vi "Get SecretKey.vi"(8 "error in (no error)":errorcluster, 11 "SMO":refnum<class "SMO.lvclass">) -> (0 "error out":errorcluster, 2 "SecretKey":string, 3 "SMO out":refnum<class "SMO.lvclass">)   [LabVIEW 2021, in "smo.lvlib" / "SMO.lvclass"]
uses:
  SMO.lvclass
  Support/Attribute.Identity/Attribute.Identity.lvclass
  SMO.lvclass/SMO.ctl
  Support/Attribute.Identity/Attribute.Identity.lvclass/Attribute.Identity.ctl
  ReftoDVR--SMO.vi
panel:
  # "For instructions on how to use the JKI State Machine Objects, examples and video tutorials, visit:\nhttp://jki.net/state-machine-objects/\n\nJKI State Machine Objects™\nhttp://jki.net/state-machine-objects/\nCopyright (C) 2005-2015, JKI <info@jki.net>\nALL RIGHTS RESERVED"
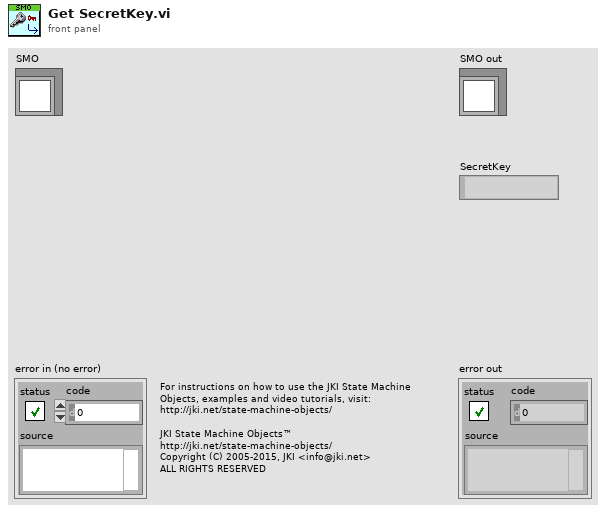
[diagram p1: front panel]
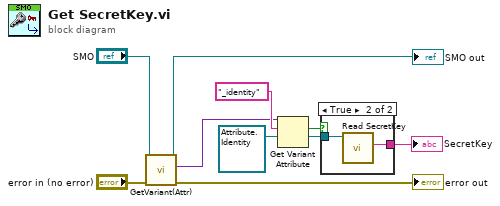
[diagram p0: block diagram]
diagram:
  n1 = call "GetVariant(Attr).vi"("error in (no error)"="error in (no error)", "SMO in"="SMO") -> ("error out"=→"error out":errorcluster, "[Attributes]"=w4:variant, "SMO out"=→"SMO out":refnum<class "SMO.lvclass">)  [unwired: 7 in]
  n2 = Get Variant Attribute(Variant=w4, name="_identity", default value (empty Variant)=refnum<class "Attribute.Identity.lvclass"> refnum ("Attribute.Identity.lvclass")) -> (found=w6:bool, value=w8:refnum<class "Attribute.Identity.lvclass">)  [unwired: 1 in, 2 out]
  n3 = case shown="True" w6 {
    tunnel: w8 -> [_ w12]
    tunnel: [_ w11] -> w7
    frame False {
    }
    frame True {
      n4 = call "Read SecretKey.vi"("Attribute.Identity in"=w12) -> ("SecretKey"=w11:string)  [unwired: 8 in, 2 out]
    }
  }
  "SecretKey" <- w7
